vi "OE2052_DATA Transmit.vi"(0 "Input Data":u8[](array[numeric])) -> (1 "Parameter Values":T2, 2 "Total Data Array":dbl[][](array[numeric]), 3 "A&B_PLL&Overload":T1)   [LabVIEW 2011]
panel:
  out "AUXIN 4_ADC":dbl
  out "AUXIN 2_ADC":dbl
  out "AUXIN 3_ADC":dbl
  out "AUXIN 1_ADC":dbl
  out "SIGIN 2_LF ADC":i32[](array[numeric])
  out "SIGIN 1_LF ADC":i32[](array[numeric])
  out "SIGIN 2_ ADC":i16[](array[numeric])
  out "SIGIN 1_ADC":i16[](array[numeric])
  out "Demod 2_X_Noise":dbl[](array[numeric])
  out "Demod 1_X_Noise":dbl[](array[numeric])
  out "Demod 4_X":dbl[](array[numeric])
  out "Demod 4_Y":dbl[](array[numeric])
  out "Demod 4_R":dbl[](array[numeric])
  out "Demod 4_Xita":dbl[](array[numeric])
  out "Demod 4_Freq":dbl[](array[numeric])
  out "Demod 3_X":dbl[](array[numeric])
  out "Demod 3_Y":dbl[](array[numeric])
  out "Demod 3_R":dbl[](array[numeric])
  out "Demod 3_Xita":dbl[](array[numeric])
  out "Demod 3_Freq":dbl[](array[numeric])
  out "B_Overload":u8
  out "B_PLL":u8
  out "A_Overload":u8
  out "A_PLL":u8
  out "Demod 1_X":dbl[](array[numeric])
  out "Demod 1_Y":dbl[](array[numeric])
  out "Demod 1_R":dbl[](array[numeric])
  out "Demod 1_Xita":dbl[](array[numeric])
  out "Demod 2_X":dbl[](array[numeric])
  out "Demod 2_Y":dbl[](array[numeric])
  out "Demod 2_R":dbl[](array[numeric])
  out "Demod 2_Xita":dbl[](array[numeric])
  out "Demod 2_Freq":dbl[](array[numeric])
  out "Demod 1_Freq":dbl[](array[numeric])
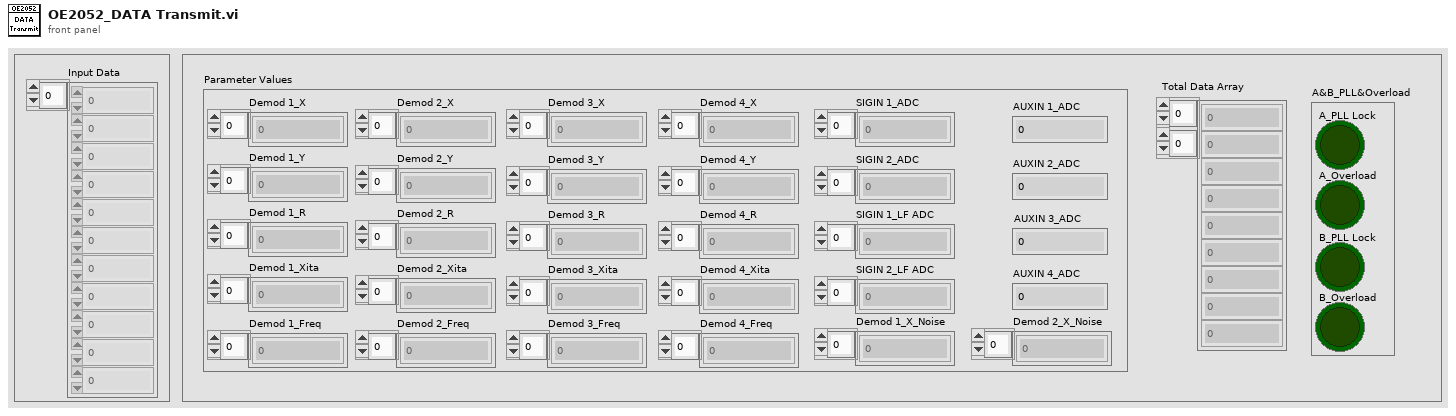
[diagram p1: front panel]
types:
  T1 = cluster{"A_PLL Lock":bool, "A_Overload":bool, "B_PLL Lock":bool, "B_Overload":bool}
  T2 = cluster{"Demod 1_X":dbl[], "Demod 1_Y":dbl[], "Demod 1_R":dbl[], "Demod 1_Xita":dbl[], "Demod 1_Freq":dbl[], "Demod 2_X":dbl[], "Demod 2_Y":dbl[], "Demod 2_R":dbl[], "Demod 2_Xita":dbl[], "Demod 2_Freq":dbl[], "Demod 3_X":dbl[], "Demod 3_Y":dbl[], "Demod 3_R":dbl[], "Demod 3_Xita":dbl[], "Demod 3_Freq":dbl[], "Demod 4_X":dbl[], "Demod 4_Y":dbl[], "Demod 4_R":dbl[], "Demod 4_Xita":dbl[], "Demod 4_Freq":dbl[], "SIGIN 1_ADC":dbl[], "SIGIN 2_ADC":dbl[], "SIGIN 1_LF ADC":dbl[], "SIGIN 2_LF ADC":dbl[], "AUXIN 1_ADC":dbl, "AUXIN 2_ADC":dbl, "AUXIN 3_ADC":dbl, "AUXIN 4_ADC":dbl, "Demod 1_X_Noise":dbl[], "Demod 2_X_Noise":dbl[]}
  T3 = cluster{"Demod 1_X":dbl[], "Demod 1_Y":dbl[], "Demod 1_R":dbl[], "Demod 1_Xita":dbl[], "Demod 1_Freq":dbl[], "Demod 2_X":dbl[], "Demod 2_Y":dbl[], "Demod 2_R":dbl[], "Demod 2_Xita":dbl[], "Demod 2_Freq":dbl[], "Demod 3_X":dbl[], "Demod 3_Y":dbl[], "Demod 3_R":dbl[], "Demod 3_Xita":dbl[], "Demod 3_Freq":dbl[], "Demod 4_X":dbl[], "Demod 4_Y":dbl[], "Demod 4_R":dbl[], "Demod 4_Xita":dbl[], "Demod 4_Freq":dbl[], "SIGIN 1_ADC":i16[], "SIGIN 2_ ADC":i16[], "SIGIN 1_LF ADC":i32[], "SIGIN 2_LF ADC":i32[], "AUXIN 1_ADC":dbl, "AUXIN 2_ADC":dbl, "AUXIN 3_ADC":dbl, "AUXIN 4_ADC":dbl, "Demod 1_X_Noise":dbl[], "Demod 2_X_Noise":dbl[]}
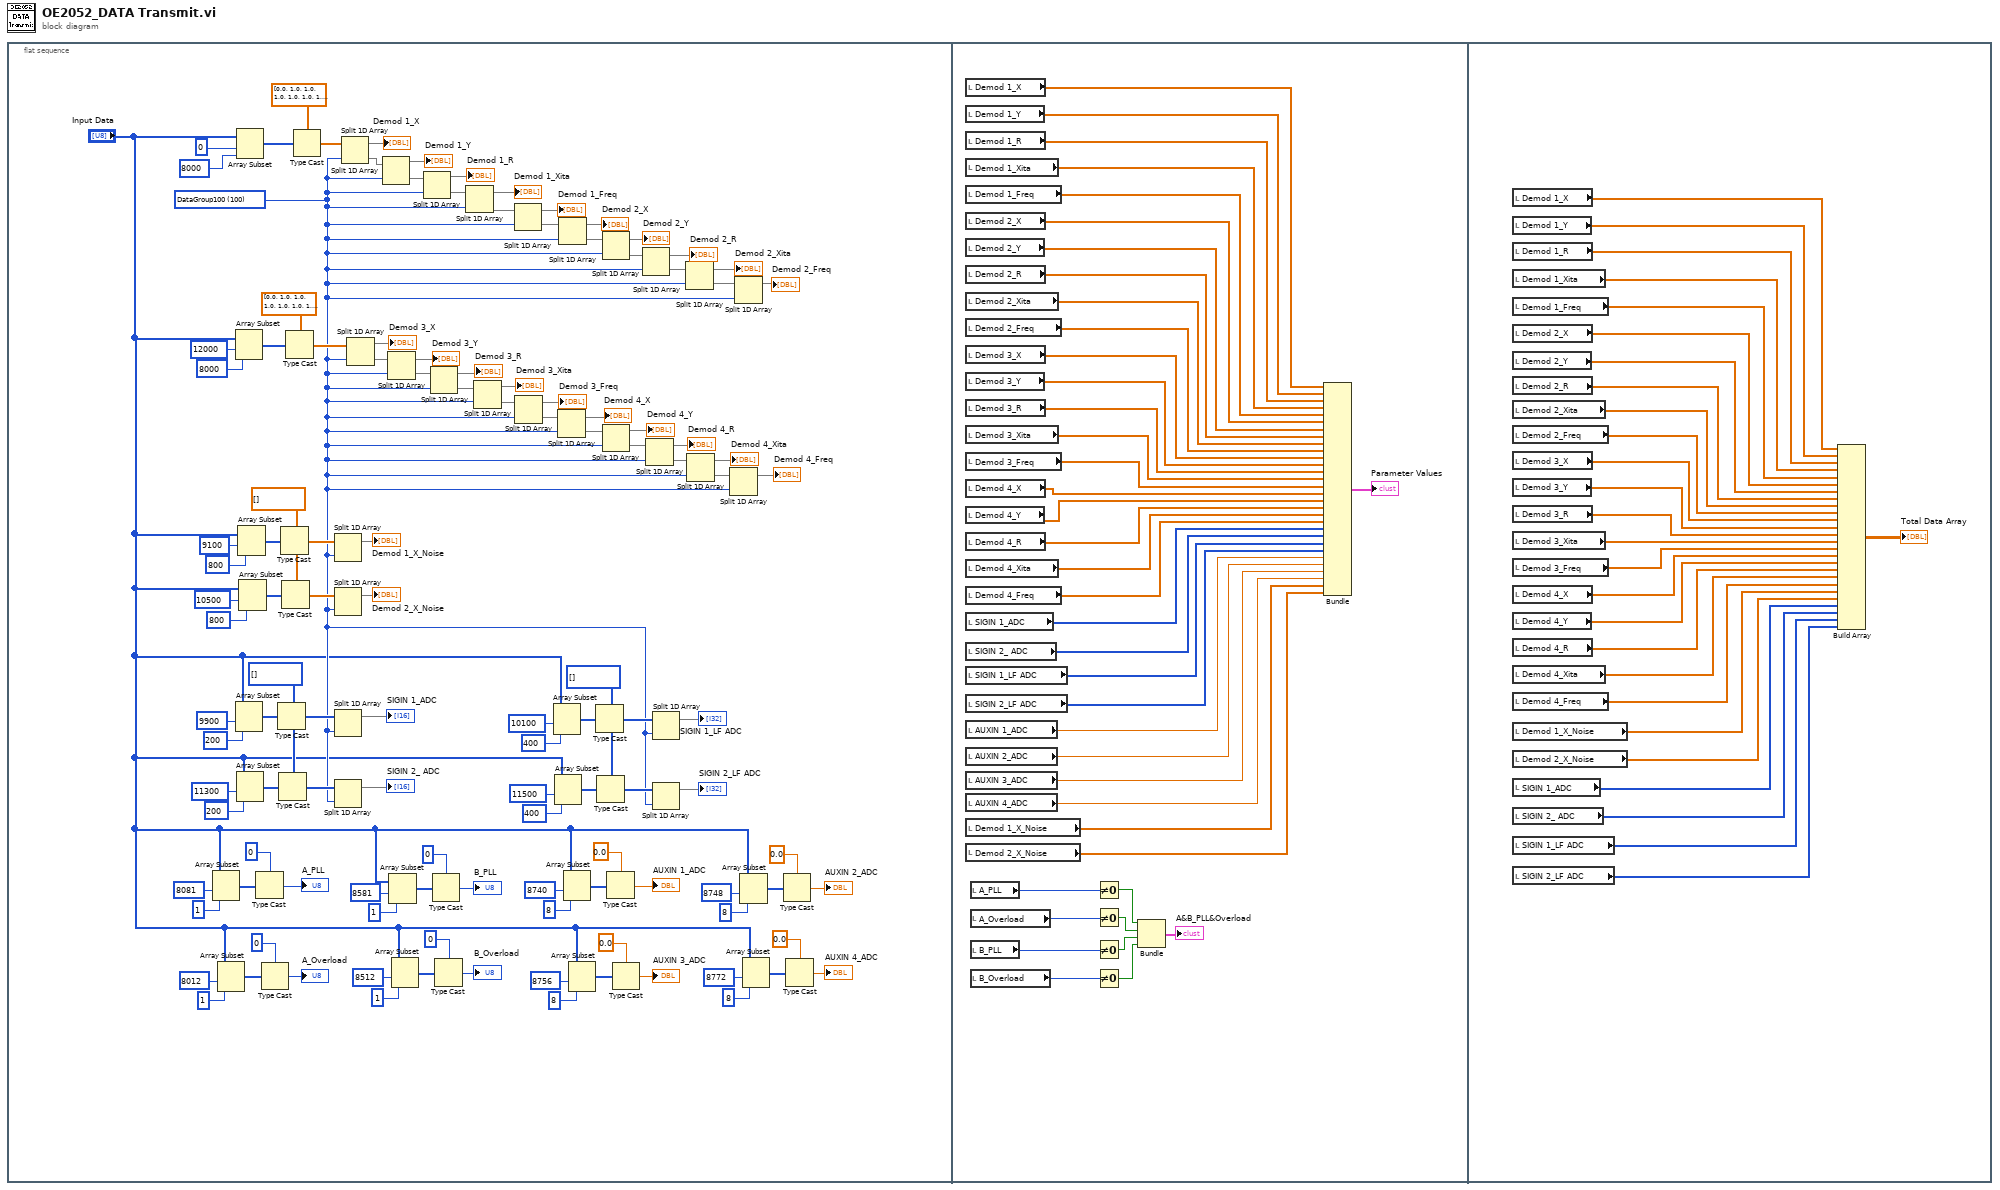
[diagram p0: block diagram]
diagram:
  n1 = flat-sequence {
    frame #0 {
      w27 = i32[] []
      w38 = i16[] []
      w49 = dbl[] []
      w24 = u16 100 items=["unsignedInt8"=1, "unsignedInt16"=2, "unsignedInt32"=4, "unsignedInt64"=8, "Float"=80, "Double"=160, "StartLength"=2240, "DataGroup50"=50, "DataGroup100"=100, "DataGroup20"=20] ("数据类型")
      n2 = Array Subset(array="Input Data", index=8081 ("索引"), length=1 ("长度")) -> (w97:u8[])
      n3 = Array Subset(array="Input Data", index=8012 ("索引"), length=1 ("长度")) -> (w92:u8[])
      n4 = Array Subset(array="Input Data", index=12000 ("索引"), length=8000 ("长度")) -> (w60:u8[])
      n5 = Array Subset(array="Input Data", index=9900 ("索引"), length=200 ("长度")) -> (w44:u8[])
      n6 = Array Subset(array="Input Data", index=0 ("索引"), length=8000 ("长度")) -> (w120:u8[])
      n7 = Array Subset(array="Input Data", index=11300 ("索引"), length=200 ("长度")) -> (w41:u8[])
      n8 = Array Subset(array="Input Data", index=9100 ("索引"), length=800 ("长度")) -> (w55:u8[])
      n9 = Array Subset(array="Input Data", index=10500 ("索引"), length=800 ("长度")) -> (w52:u8[])
      n10 = Type Cast(type=u8 0, x=w97) -> (*(type *) &x=→"A_PLL":u8)
      n11 = Type Cast(type=u8 0, x=w92) -> (*(type *) &x=→"A_Overload":u8)
      n12 = Type Cast(type=w38, x=w44) -> (*(type *) &x=w37:i16[])
      n13 = Type Cast(type=w38, x=w41) -> (*(type *) &x=w36:i16[])
      n14 = Type Cast(type=w49, x=w55) -> (*(type *) &x=w48:dbl[])
      n15 = Type Cast(type=w49, x=w52) -> (*(type *) &x=w47:dbl[])
      n16 = Type Cast(type=dbl[] [0.0, 1.0, 1.0, 1.0, 1.0, 1.0, 1.0, 1.0, 1.0, 1.0, 1.0, 1.0, 1.0, 1.0, 1.0, 1.0, 1.0, 1.0, 1.0, 1.0, 1.0, 1.0, 1.0, 1.0, 1.0, 1.0, 1.0, 1.0, 1.0, 1.0, 1.0, 1.0, 1.0, 1.0, 1.0, 1.0, 1.0, 1.0, 1.0, 1.0, 1.0, 1.0, 1.0, 1.0, 1.0, 1.0, 1.0, 1.0, 1.0, 1.0, 1.0, 1.0, 1.0, 1.0, 1.0, 1.0, 1.0, 1.0, 1.0, 1.0, 1.0, 1.0, 1.0, 1.0, 1.0, 1.0, 1.0, 1.0, 1.0, 1.0, 1.0, 1.0, 1.0, 1.0, 1.0, 1.0, 1.0, 1.0, 1.0, 1.0, 1.0, 1.0, 1.0, 1.0, 1.0, 1.0, 1.0, 1.0, 1.0, 1.0, 1.0, 1.0, 1.0, 1.0, 1.0, 1.0, 1.0, 1.0, 1.0, 1.0, 1.0, 1.0, 1.0, 1.0, 1.0, 1.0, 1.0, 1.0, 1.0, 1.0, 1.0, 1.0, 1.0, 1.0, 1.0, 1.0, 1.0, 1.0, 1.0, 1.0, 1.0, 1.0, 1.0, 1.0, 1.0, 1.0, 1.0, 1.0, 1.0, 1.0, 1.0, 1.0, 1.0, 1.0, 1.0, 1.0, 1.0, 1.0, 1.0, 1.0, 1.0, 1.0, 1.0, 1.0, 1.0, 1.0, 1.0, 1.0, 1.0, 1.0, 1.0, 1.0, 1.0, 1.0, 1.0, 1.0, 1.0, 1.0, 1.0, 1.0, 1.0, 1.0, 1.0, 1.0, 1.0, 1.0, 1.0, 1.0, 1.0, 1.0, 1.0, 1.0, 1.0, 1.0, 1.0, 1.0, 1.0, 1.0, 1.0, 1.0, 1.0, 1.0, 1.0, 1.0, 1.0, 1.0, 1.0, 1.0, 1.0, 1.0, 1.0, 1.0, 1.0, 1.0, 1.0, 1.0, 1.0, 1.0, 1.0, 1.0, 1.0, 1.0, 1.0, 1.0, 1.0, 1.0, 1.0, 1.0, 1.0, 1.0, 1.0, 1.0, 1.0, 1.0, 1.0, 1.0, 1.0, 1.0, 1.0, 1.0, 1.0, 1.0, 1.0, 1.0, 1.0, 1.0, 1.0, 1.0, 1.0, 1.0, 1.0, 1.0, 1.0, 1.0, 1.0, 1.0, 1.0, 1.0, 1.0, 1.0, 1.0, 1.0, 1.0, 1.0, 1.0, 1.0, 1.0, 1.0, 1.0, 1.0, 1.0, 1.0, 1.0, 1.0, 1.0, 1.0, 1.0, 1.0, 1.0, 1.0, 1.0, 1.0, 1.0, 1.0, 1.0, 1.0, 1.0, 1.0, 1.0, 1.0, 1.0, 1.0, 1.0, 1.0, 1.0, 1.0, 1.0, 1.0, 1.0, 1.0, 1.0, 1.0, 1.0, 1.0, 1.0, 1.0, 1.0, 1.0, 1.0, 1.0, 1.0, 1.0, 1.0, 1.0, 1.0, 1.0, 1.0, 1.0, 1.0, 1.0, 1.0, 1.0, 1.0, 1.0, 1.0, 1.0, 1.0, 1.0, 1.0, 1.0, 1.0, 1.0, 1.0, 1.0, 1.0, 1.0, 1.0, 1.0, 1.0, 1.0, 1.0, 1.0, 1.0, 1.0, 1.0, 1.0, 1.0, 1.0, 1.0, 1.0, 1.0, 1.0, 1.0, 1.0, 1.0, 1.0, 1.0, 1.0, 1.0, 1.0, 1.0, 1.0, 1.0, 1.0, 1.0, 1.0, 1.0, 1.0, 1.0, 1.0, 1.0, 1.0, 1.0, 1.0, 1.0, 1.0, 1.0, 1.0, 1.0, 1.0, 1.0, 1.0, 1.0, 1.0, 1.0, 1.0, 1.0, 1.0, 1.0, 1.0, 1.0, 1.0, 1.0, 1.0, 1.0, 1.0, 1.0, 1.0, 1.0, 1.0, 1.0, 1.0, 1.0, 1.0, 1.0, 1.0, 1.0, 1.0, 1.0, 1.0, 1.0, 1.0, 1.0, 1.0, 1.0, 1.0, 1.0, 1.0, 1.0, 1.0, 0.0, 1.0, 1.0, 1.0, 1.0, 1.0, 1.0, 1.0, 1.0, 1.0, 1.0, 1.0, 1.0, 1.0, 1.0, 1.0, 1.0, 1.0, 1.0, 1.0, 1.0, 1.0, 1.0, 1.0, 1.0, 1.0, 1.0, 1.0, 1.0, 1.0, 1.0, 1.0, 1.0, 1.0, 1.0, 1.0, 1.0, 1.0, 1.0, 1.0, 1.0, 1.0, 1.0, 1.0, 1.0, 1.0, 1.0, 1.0, 1.0, 1.0, 1.0, 1.0, 1.0, 1.0, 1.0, 1.0, 1.0, 1.0, 1.0, 1.0, 1.0, 1.0, 1.0, 1.0, 1.0, 1.0, 1.0, 1.0, 1.0, 1.0, 1.0, 1.0, 1.0, 1.0, 1.0, 1.0, 1.0, 1.0, 1.0, 1.0, 1.0, 1.0, 1.0, 1.0, 1.0, 1.0, 1.0, 1.0, 1.0, 1.0, 1.0, 1.0, 1.0, 1.0, 1.0, 1.0, 1.0, 1.0, 1.0, 1.0, 1.0, 1.0, 1.0, 1.0, 1.0, 1.0, 1.0, 1.0, 1.0, 1.0, 1.0, 1.0, 1.0, 1.0, 1.0, 1.0, 1.0, 1.0, 1.0, 1.0, 1.0, 1.0, 1.0, 1.0, 1.0, 1.0, 1.0, 1.0, 1.0, 1.0, 1.0, 1.0, 1.0, 1.0, 1.0, 1.0, 1.0, 1.0, 1.0, 1.0, 1.0, 1.0, 1.0, 1.0, 1.0, 1.0, 1.0, 1.0, 1.0, 1.0, 1.0, 1.0, 1.0, 1.0, 1.0, 1.0, 1.0, 1.0, 1.0, 1.0, 1.0, 1.0, 1.0, 1.0, 1.0, 1.0, 1.0, 1.0, 1.0, 1.0, 1.0, 1.0, 1.0, 1.0, 1.0, 1.0, 1.0, 1.0, 1.0, 1.0, 1.0, 1.0, 1.0, 1.0, 1.0, 1.0, 1.0, 1.0, 1.0, 1.0, 1.0, 1.0, 1.0, 1.0, 1.0, 1.0, 1.0, 1.0, 1.0, 1.0, 1.0, 1.0, 1.0, 1.0, 1.0, 1.0, 1.0, 1.0, 1.0, 1.0, 1.0, 1.0, 1.0, 1.0, 1.0, 1.0, 1.0, 1.0, 1.0, 1.0, 1.0, 1.0, 1.0, 1.0, 1.0, 1.0, 1.0, 1.0, 1.0, 1.0, 1.0, 1.0, 1.0, 1.0, 1.0, 1.0, 1.0, 1.0, 1.0, 1.0, 1.0, 1.0, 1.0, 1.0, 1.0, 1.0, 1.0, 1.0, 1.0, 1.0, 1.0, 1.0, 1.0, 1.0, 1.0, 1.0, 1.0, 1.0, 1.0, 1.0, 1.0, 1.0, 1.0, 1.0, 1.0, 1.0, 1.0, 1.0, 1.0, 1.0, 1.0, 1.0, 1.0, 1.0, 1.0, 1.0, 1.0, 1.0, 1.0, 1.0, 1.0, 1.0, 1.0, 1.0, 1.0, 1.0, 1.0, 1.0, 1.0, 1.0, 1.0, 1.0, 1.0, 1.0, 1.0, 1.0, 1.0, 1.0, 1.0, 1.0, 1.0, 1.0, 1.0, 1.0, 1.0, 1.0, 1.0, 1.0, 1.0, 1.0, 1.0, 1.0, 1.0, 1.0, 1.0, 1.0, 1.0, 1.0, 1.0, 1.0, 1.0, 1.0, 1.0, 1.0, 1.0, 1.0, 1.0, 1.0, 1.0, 1.0, 1.0, 1.0, 1.0, 1.0, 1.0, 1.0, 1.0, 1.0, 1.0, 1.0, 1.0, 1.0, 1.0, 1.0, 1.0, 1.0, 1.0, 1.0, 1.0, 1.0, 1.0, 1.0, 1.0, 1.0, 1.0, 1.0, 1.0, 1.0, 1.0, 1.0, 1.0, 1.0, 1.0, 1.0, 1.0, 1.0, 1.0, 1.0, 1.0, 1.0, 1.0, 1.0, 1.0, 1.0, 1.0, 1.0, 1.0, 1.0, 1.0, 1.0, 1.0, 1.0, 1.0, 1.0, 1.0, 1.0, 1.0, 1.0, 1.0, 1.0, 1.0, 1.0, 1.0, 1.0, 1.0, 1.0, 1.0, 1.0, 1.0, 1.0], x=w60) -> (*(type *) &x=w57:dbl[])
      n17 = Type Cast(type=dbl[] [0.0, 1.0, 1.0, 1.0, 1.0, 1.0, 1.0, 1.0, 1.0, 1.0, 1.0, 1.0, 1.0, 1.0, 1.0, 1.0, 1.0, 1.0, 1.0, 1.0, 1.0, 1.0, 1.0, 1.0, 1.0, 1.0, 1.0, 1.0, 1.0, 1.0, 1.0, 1.0, 1.0, 1.0, 1.0, 1.0, 1.0, 1.0, 1.0, 1.0, 1.0, 1.0, 1.0, 1.0, 1.0, 1.0, 1.0, 1.0, 1.0, 1.0, 1.0, 1.0, 1.0, 1.0, 1.0, 1.0, 1.0, 1.0, 1.0, 1.0, 1.0, 1.0, 1.0, 1.0, 1.0, 1.0, 1.0, 1.0, 1.0, 1.0, 1.0, 1.0, 1.0, 1.0, 1.0, 1.0, 1.0, 1.0, 1.0, 1.0, 1.0, 1.0, 1.0, 1.0, 1.0, 1.0, 1.0, 1.0, 1.0, 1.0, 1.0, 1.0, 1.0, 1.0, 1.0, 1.0, 1.0, 1.0, 1.0, 1.0, 1.0, 1.0, 1.0, 1.0, 1.0, 1.0, 1.0, 1.0, 1.0, 1.0, 1.0, 1.0, 1.0, 1.0, 1.0, 1.0, 1.0, 1.0, 1.0, 1.0, 1.0, 1.0, 1.0, 1.0, 1.0, 1.0, 1.0, 1.0, 1.0, 1.0, 1.0, 1.0, 1.0, 1.0, 1.0, 1.0, 1.0, 1.0, 1.0, 1.0, 1.0, 1.0, 1.0, 1.0, 1.0, 1.0, 1.0, 1.0, 1.0, 1.0, 1.0, 1.0, 1.0, 1.0, 1.0, 1.0, 1.0, 1.0, 1.0, 1.0, 1.0, 1.0, 1.0, 1.0, 1.0, 1.0, 1.0, 1.0, 1.0, 1.0, 1.0, 1.0, 1.0, 1.0, 1.0, 1.0, 1.0, 1.0, 1.0, 1.0, 1.0, 1.0, 1.0, 1.0, 1.0, 1.0, 1.0, 1.0, 1.0, 1.0, 1.0, 1.0, 1.0, 1.0, 1.0, 1.0, 1.0, 1.0, 1.0, 1.0, 1.0, 1.0, 1.0, 1.0, 1.0, 1.0, 1.0, 1.0, 1.0, 1.0, 1.0, 1.0, 1.0, 1.0, 1.0, 1.0, 1.0, 1.0, 1.0, 1.0, 1.0, 1.0, 1.0, 1.0, 1.0, 1.0, 1.0, 1.0, 1.0, 1.0, 1.0, 1.0, 1.0, 1.0, 1.0, 1.0, 1.0, 1.0, 1.0, 1.0, 1.0, 1.0, 1.0, 1.0, 1.0, 1.0, 1.0, 1.0, 1.0, 1.0, 1.0, 1.0, 1.0, 1.0, 1.0, 1.0, 1.0, 1.0, 1.0, 1.0, 1.0, 1.0, 1.0, 1.0, 1.0, 1.0, 1.0, 1.0, 1.0, 1.0, 1.0, 1.0, 1.0, 1.0, 1.0, 1.0, 1.0, 1.0, 1.0, 1.0, 1.0, 1.0, 1.0, 1.0, 1.0, 1.0, 1.0, 1.0, 1.0, 1.0, 1.0, 1.0, 1.0, 1.0, 1.0, 1.0, 1.0, 1.0, 1.0, 1.0, 1.0, 1.0, 1.0, 1.0, 1.0, 1.0, 1.0, 1.0, 1.0, 1.0, 1.0, 1.0, 1.0, 1.0, 1.0, 1.0, 1.0, 1.0, 1.0, 1.0, 1.0, 1.0, 1.0, 1.0, 1.0, 1.0, 1.0, 1.0, 1.0, 1.0, 1.0, 1.0, 1.0, 1.0, 1.0, 1.0, 1.0, 1.0, 1.0, 1.0, 1.0, 1.0, 1.0, 1.0, 1.0, 1.0, 1.0, 1.0, 1.0, 1.0, 1.0, 1.0, 1.0, 1.0, 1.0, 1.0, 1.0, 1.0, 1.0, 1.0, 1.0, 1.0, 1.0, 1.0, 1.0, 1.0, 1.0, 1.0, 1.0, 1.0, 1.0, 1.0, 1.0, 1.0, 1.0, 1.0, 1.0, 1.0, 1.0, 1.0, 1.0, 1.0, 1.0, 1.0, 1.0, 1.0, 1.0, 1.0, 1.0, 1.0, 1.0, 1.0, 1.0, 1.0, 1.0, 1.0, 1.0, 1.0, 1.0, 1.0, 0.0, 1.0, 1.0, 1.0, 1.0, 1.0, 1.0, 1.0, 1.0, 1.0, 1.0, 1.0, 1.0, 1.0, 1.0, 1.0, 1.0, 1.0, 1.0, 1.0, 1.0, 1.0, 1.0, 1.0, 1.0, 1.0, 1.0, 1.0, 1.0, 1.0, 1.0, 1.0, 1.0, 1.0, 1.0, 1.0, 1.0, 1.0, 1.0, 1.0, 1.0, 1.0, 1.0, 1.0, 1.0, 1.0, 1.0, 1.0, 1.0, 1.0, 1.0, 1.0, 1.0, 1.0, 1.0, 1.0, 1.0, 1.0, 1.0, 1.0, 1.0, 1.0, 1.0, 1.0, 1.0, 1.0, 1.0, 1.0, 1.0, 1.0, 1.0, 1.0, 1.0, 1.0, 1.0, 1.0, 1.0, 1.0, 1.0, 1.0, 1.0, 1.0, 1.0, 1.0, 1.0, 1.0, 1.0, 1.0, 1.0, 1.0, 1.0, 1.0, 1.0, 1.0, 1.0, 1.0, 1.0, 1.0, 1.0, 1.0, 1.0, 1.0, 1.0, 1.0, 1.0, 1.0, 1.0, 1.0, 1.0, 1.0, 1.0, 1.0, 1.0, 1.0, 1.0, 1.0, 1.0, 1.0, 1.0, 1.0, 1.0, 1.0, 1.0, 1.0, 1.0, 1.0, 1.0, 1.0, 1.0, 1.0, 1.0, 1.0, 1.0, 1.0, 1.0, 1.0, 1.0, 1.0, 1.0, 1.0, 1.0, 1.0, 1.0, 1.0, 1.0, 1.0, 1.0, 1.0, 1.0, 1.0, 1.0, 1.0, 1.0, 1.0, 1.0, 1.0, 1.0, 1.0, 1.0, 1.0, 1.0, 1.0, 1.0, 1.0, 1.0, 1.0, 1.0, 1.0, 1.0, 1.0, 1.0, 1.0, 1.0, 1.0, 1.0, 1.0, 1.0, 1.0, 1.0, 1.0, 1.0, 1.0, 1.0, 1.0, 1.0, 1.0, 1.0, 1.0, 1.0, 1.0, 1.0, 1.0, 1.0, 1.0, 1.0, 1.0, 1.0, 1.0, 1.0, 1.0, 1.0, 1.0, 1.0, 1.0, 1.0, 1.0, 1.0, 1.0, 1.0, 1.0, 1.0, 1.0, 1.0, 1.0, 1.0, 1.0, 1.0, 1.0, 1.0, 1.0, 1.0, 1.0, 1.0, 1.0, 1.0, 1.0, 1.0, 1.0, 1.0, 1.0, 1.0, 1.0, 1.0, 1.0, 1.0, 1.0, 1.0, 1.0, 1.0, 1.0, 1.0, 1.0, 1.0, 1.0, 1.0, 1.0, 1.0, 1.0, 1.0, 1.0, 1.0, 1.0, 1.0, 1.0, 1.0, 1.0, 1.0, 1.0, 1.0, 1.0, 1.0, 1.0, 1.0, 1.0, 1.0, 1.0, 1.0, 1.0, 1.0, 1.0, 1.0, 1.0, 1.0, 1.0, 1.0, 1.0, 1.0, 1.0, 1.0, 1.0, 1.0, 1.0, 1.0, 1.0, 1.0, 1.0, 1.0, 1.0, 1.0, 1.0, 1.0, 1.0, 1.0, 1.0, 1.0, 1.0, 1.0, 1.0, 1.0, 1.0, 1.0, 1.0, 1.0, 1.0, 1.0, 1.0, 1.0, 1.0, 1.0, 1.0, 1.0, 1.0, 1.0, 1.0, 1.0, 1.0, 1.0, 1.0, 1.0, 1.0, 1.0, 1.0, 1.0, 1.0, 1.0, 1.0, 1.0, 1.0, 1.0, 1.0, 1.0, 1.0, 1.0, 1.0, 1.0, 1.0, 1.0, 1.0, 1.0, 1.0, 1.0, 1.0, 1.0, 1.0, 1.0, 1.0, 1.0, 1.0, 1.0, 1.0, 1.0, 1.0, 1.0, 1.0, 1.0, 1.0, 1.0, 1.0, 1.0, 1.0, 1.0, 1.0, 1.0, 1.0, 1.0, 1.0, 1.0, 1.0, 1.0, 1.0, 1.0, 1.0, 1.0, 1.0, 1.0, 1.0, 1.0, 1.0, 1.0, 1.0, 1.0, 1.0, 1.0, 1.0, 1.0, 1.0, 1.0, 1.0, 1.0, 1.0, 1.0, 1.0, 1.0, 1.0, 1.0, 1.0, 1.0, 1.0, 1.0, 1.0], x=w120) -> (*(type *) &x=w115:dbl[])
      n18 = Split 1D Array(array=w48, index=w24) -> (first subarray=→"Demod 1_X_Noise":dbl[])  [unwired: 1 out]
      n19 = Split 1D Array(array=w47, index=w24) -> (first subarray=→"Demod 2_X_Noise":dbl[])  [unwired: 1 out]
      n20 = Split 1D Array(array=w37, index=w24) -> (first subarray=→"SIGIN 1_ADC":i16[])  [unwired: 1 out]
      n21 = Split 1D Array(array=w36, index=w24) -> (first subarray=→"SIGIN 2_ ADC":i16[])  [unwired: 1 out]
      n22 = Split 1D Array(array=w115, index=w24) -> (first subarray=→"Demod 1_X":dbl[], second subarray=w116:dbl[])
      n23 = Split 1D Array(array=w57, index=w24) -> (first subarray=→"Demod 3_X":dbl[], second subarray=w77:dbl[])
      n24 = Split 1D Array(array=w116, index=w24) -> (first subarray=→"Demod 1_Y":dbl[], second subarray=w121:dbl[])
      n25 = Split 1D Array(array=w77, index=w24) -> (first subarray=→"Demod 3_Y":dbl[], second subarray=w79:dbl[])
      n26 = Array Subset(array="Input Data", index=8581 ("索引"), length=1 ("长度")) -> (w87:u8[])
      n27 = Array Subset(array="Input Data", index=8512 ("索引"), length=1 ("长度")) -> (w82:u8[])
      n28 = Split 1D Array(array=w121, index=w24) -> (first subarray=→"Demod 1_R":dbl[], second subarray=w108:dbl[])
      n29 = Split 1D Array(array=w79, index=w24) -> (first subarray=→"Demod 3_R":dbl[], second subarray=w76:dbl[])
      n30 = Type Cast(type=u8 0, x=w87) -> (*(type *) &x=→"B_PLL":u8)
      n31 = Type Cast(type=u8 0, x=w82) -> (*(type *) &x=→"B_Overload":u8)
      n32 = Split 1D Array(array=w108, index=w24) -> (first subarray=→"Demod 1_Xita":dbl[], second subarray=w110:dbl[])
      n33 = Split 1D Array(array=w76, index=w24) -> (first subarray=→"Demod 3_Xita":dbl[], second subarray=w75:dbl[])
      n34 = Split 1D Array(array=w110, index=w24) -> (first subarray=→"Demod 1_Freq":dbl[], second subarray=w109:dbl[])
      n35 = Split 1D Array(array=w75, index=w24) -> (first subarray=→"Demod 3_Freq":dbl[], second subarray=w78:dbl[])
      n36 = Array Subset(array="Input Data", index=10100 ("索引"), length=400 ("长度")) -> (w33:u8[])
      n37 = Array Subset(array="Input Data", index=11500 ("索引"), length=400 ("长度")) -> (w30:u8[])
      n38 = Split 1D Array(array=w78, index=w24) -> (first subarray=→"Demod 4_X":dbl[], second subarray=w71:dbl[])
      n39 = Split 1D Array(array=w109, index=w24) -> (first subarray=→"Demod 2_X":dbl[], second subarray=w119:dbl[])
      n40 = Array Subset(array="Input Data", index=8740 ("索引"), length=8 ("长度")) -> (w19:u8[])
      n41 = Array Subset(array="Input Data", index=8756 ("索引"), length=8 ("长度")) -> (w14:u8[])
      n42 = Type Cast(type=w27, x=w33) -> (*(type *) &x=w26:i32[])
      n43 = Type Cast(type=w27, x=w30) -> (*(type *) &x=w25:i32[])
      n44 = Split 1D Array(array=w119, index=w24) -> (first subarray=→"Demod 2_Y":dbl[], second subarray=w122:dbl[])
      n45 = Split 1D Array(array=w71, index=w24) -> (first subarray=→"Demod 4_Y":dbl[], second subarray=w73:dbl[])
      n46 = Type Cast(type=0.0, x=w19) -> (*(type *) &x=→"AUXIN 1_ADC":dbl)
      n47 = Type Cast(type=0.0, x=w14) -> (*(type *) &x=→"AUXIN 3_ADC":dbl)
      n48 = Split 1D Array(array=w122, index=w24) -> (first subarray=→"Demod 2_R":dbl[], second subarray=w123:dbl[])
      n49 = Split 1D Array(array=w73, index=w24) -> (first subarray=→"Demod 4_R":dbl[], second subarray=w72:dbl[])
      n50 = Split 1D Array(array=w26, index=w24) -> (first subarray=→"SIGIN 1_LF ADC":i32[])  [unwired: 1 out]
      n51 = Split 1D Array(array=w25, index=w24) -> (first subarray=→"SIGIN 2_LF ADC":i32[])  [unwired: 1 out]
      n52 = Split 1D Array(array=w123, index=w24) -> (first subarray=→"Demod 2_Xita":dbl[], second subarray=w112:dbl[])
      n53 = Split 1D Array(array=w72, index=w24) -> (first subarray=→"Demod 4_Xita":dbl[], second subarray=w74:dbl[])
      n54 = Split 1D Array(array=w74, index=w24) -> (first subarray=→"Demod 4_Freq":dbl[])  [unwired: 1 out]
      n55 = Split 1D Array(array=w112, index=w24) -> (first subarray=→"Demod 2_Freq":dbl[])  [unwired: 1 out]
      n56 = Array Subset(array="Input Data", index=8748 ("索引"), length=8 ("长度")) -> (w9:u8[])
      n57 = Array Subset(array="Input Data", index=8772 ("索引"), length=8 ("长度")) -> (w4:u8[])
      n58 = Type Cast(type=0.0, x=w9) -> (*(type *) &x=→"AUXIN 2_ADC":dbl)
      n59 = Type Cast(type=0.0, x=w4) -> (*(type *) &x=→"AUXIN 4_ADC":dbl)
    }
    frame #1 {
      n60 = local read "Demod 1_X"() -> (w163:dbl[])
      n61 = local read "Demod 1_Y"() -> (w162:dbl[])
      n62 = local read "Demod 1_R"() -> (w161:dbl[])
      n63 = local read "Demod 1_Xita"() -> (w160:dbl[])
      n64 = local read "Demod 1_Freq"() -> (w159:dbl[])
      n65 = local read "Demod 2_X"() -> (w158:dbl[])
      n66 = local read "Demod 2_Y"() -> (w157:dbl[])
      n67 = local read "Demod 2_R"() -> (w156:dbl[])
      n68 = local read "Demod 2_Xita"() -> (w155:dbl[])
      n69 = local read "Demod 2_Freq"() -> (w154:dbl[])
      n70 = local read "Demod 3_X"() -> (w144:dbl[])
      n71 = local read "Demod 3_Y"() -> (w143:dbl[])
      n72 = local read "Demod 3_R"() -> (w142:dbl[])
      n73 = local read "Demod 3_Xita"() -> (w141:dbl[])
      n74 = local read "Demod 3_Freq"() -> (w135:dbl[])
      n75 = local read "Demod 4_X"() -> (w140:dbl[])
      n76 = local read "Demod 4_Y"() -> (w139:dbl[])
      n77 = local read "Demod 4_R"() -> (w138:dbl[])
      n78 = local read "Demod 4_Xita"() -> (w137:dbl[])
      n79 = local read "Demod 4_Freq"() -> (w136:dbl[])
      n80 = local read "SIGIN 1_ADC"() -> (w134:i16[])
      n81 = local read "SIGIN 2_ ADC"() -> (w133:i16[])
      n82 = local read "SIGIN 1_LF ADC"() -> (w132:i32[])
      n83 = local read "SIGIN 2_LF ADC"() -> (w131:i32[])
      n84 = local read "AUXIN 1_ADC"() -> (w130:dbl)
      n85 = local read "AUXIN 2_ADC"() -> (w129:dbl)
      n86 = local read "AUXIN 3_ADC"() -> (w128:dbl)
      n87 = local read "AUXIN 4_ADC"() -> (w127:dbl)
      n88 = local read "Demod 1_X_Noise"() -> (w126:dbl[])
      n89 = local read "Demod 2_X_Noise"() -> (w125:dbl[])
      n90 = local read "A_PLL"() -> (w147:u8)
      n91 = local read "A_Overload"() -> (w148:u8)
      n92 = local read "B_PLL"() -> (w149:u8)
      n93 = local read "B_Overload"() -> (w150:u8)
      n94 = Not Equal To 0?(x=w147) -> (x != 0?=w152:bool)
      n95 = Not Equal To 0?(x=w148) -> (x != 0?=w153:bool)
      n96 = Not Equal To 0?(x=w149) -> (x != 0?=w151:bool)
      n97 = Not Equal To 0?(x=w150) -> (x != 0?=w146:bool)
      n98 = Bundle(w152, w153, w151, w146) -> (→"A&B_PLL&Overload":cluster{bool, bool, bool, bool})  [unwired: 1 in]
      n99 = Bundle("Demod 1_X"=w163, "Demod 1_Y"=w162, "Demod 1_R"=w161, "Demod 1_Xita"=w160, "Demod 1_Freq"=w159, "Demod 2_X"=w158, "Demod 2_Y"=w157, "Demod 2_R"=w156, "Demod 2_Xita"=w155, "Demod 2_Freq"=w154, "Demod 3_X"=w144, "Demod 3_Y"=w143, "Demod 3_R"=w142, "Demod 3_Xita"=w141, "Demod 3_Freq"=w135, "Demod 4_X"=w140, "Demod 4_Y"=w139, "Demod 4_R"=w138, "Demod 4_Xita"=w137, "Demod 4_Freq"=w136, "SIGIN 1_ADC"=w134, "SIGIN 2_ ADC"=w133, "SIGIN 1_LF ADC"=w132, "SIGIN 2_LF ADC"=w131, "AUXIN 1_ADC"=w130, "AUXIN 2_ADC"=w129, "AUXIN 3_ADC"=w128, "AUXIN 4_ADC"=w127, "Demod 1_X_Noise"=w126, "Demod 2_X_Noise"=w125) -> (→"Parameter Values":T3)  [unwired: 1 in]
    }
    frame #2 {
      n100 = local read "Demod 1_X"() -> (w183:dbl[])
      n101 = local read "Demod 1_Y"() -> (w184:dbl[])
      n102 = local read "Demod 1_R"() -> (w185:dbl[])
      n103 = local read "Demod 1_Xita"() -> (w186:dbl[])
      n104 = local read "Demod 1_Freq"() -> (w187:dbl[])
      n105 = local read "Demod 2_X"() -> (w188:dbl[])
      n106 = local read "Demod 2_Y"() -> (w189:dbl[])
      n107 = local read "Demod 2_R"() -> (w190:dbl[])
      n108 = local read "Demod 2_Xita"() -> (w180:dbl[])
      n109 = local read "Demod 2_Freq"() -> (w181:dbl[])
      n110 = local read "Demod 3_X"() -> (w179:dbl[])
      n111 = local read "Demod 3_Y"() -> (w178:dbl[])
      n112 = local read "Demod 3_R"() -> (w177:dbl[])
      n113 = local read "Demod 3_Xita"() -> (w176:dbl[])
      n114 = local read "Demod 3_Freq"() -> (w175:dbl[])
      n115 = local read "Demod 4_X"() -> (w174:dbl[])
      n116 = local read "Demod 4_Y"() -> (w173:dbl[])
      n117 = local read "Demod 4_R"() -> (w172:dbl[])
      n118 = local read "Demod 4_Xita"() -> (w171:dbl[])
      n119 = local read "Demod 4_Freq"() -> (w170:dbl[])
      n120 = local read "Demod 1_X_Noise"() -> (w169:dbl[])
      n121 = local read "Demod 2_X_Noise"() -> (w164:dbl[])
      n122 = local read "SIGIN 1_ADC"() -> (w168:i16[])
      n123 = local read "SIGIN 2_ ADC"() -> (w167:i16[])
      n124 = local read "SIGIN 1_LF ADC"() -> (w166:i32[])
      n125 = local read "SIGIN 2_LF ADC"() -> (w165:i32[])
      n126 = Build Array(w183, w184, w185, w186, w187, w188, w189, w190, w180, w181, w179, w178, w177, w176, w175, w174, w173, w172, w171, w170, w169, w164, w168, w167, w166, w165) -> (→"Total Data Array":dbl[][])
    }
  }
